vi "Demo.vi"() -> ()   [LabVIEW 2011, in "Mlistbox Tools.lvlib"]
uses:
  Mlistbox Tools.lvlib
  ListBox/Custom Type/Read and Write Mode.ctl
  ListBox/Listbox Tool.lvlib
  Custom Type/Row and Col Option.ctl
panel:
  out "数值显示控件":dbl
  in  "多列列表框":i32(listbox)
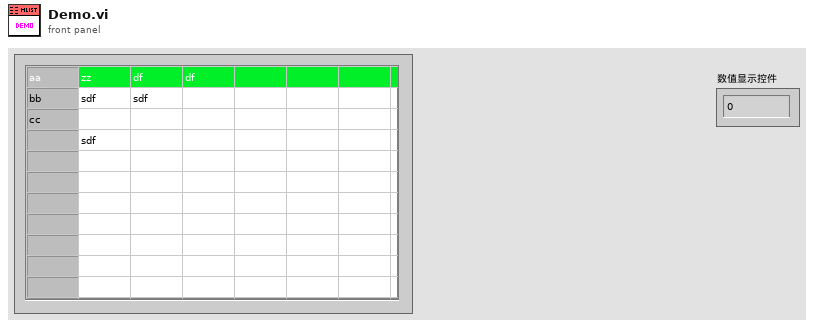
[diagram p1: front panel]
types:
  T1 = typedef "Mlistbox Tools.lvlib/Row and Col Option.ctl" = enum16{"Row", "Col"}
  T2 = typedef "Listbox Tool.lvlib/Read and Write Mode.ctl" = enum16{"Read", "Write"}
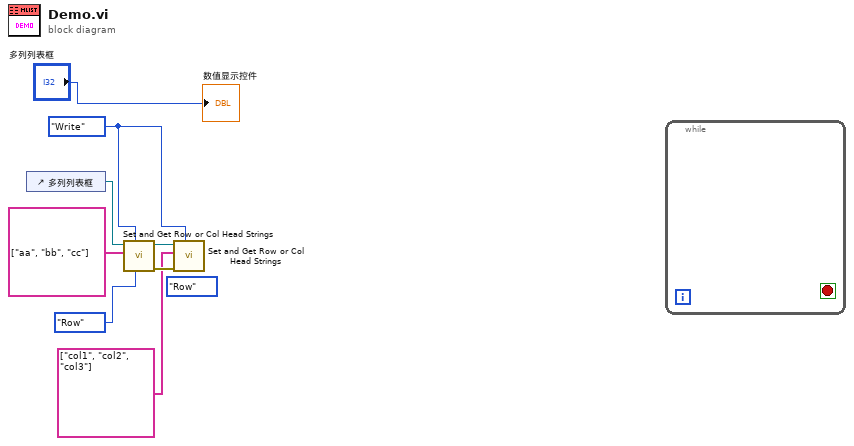
[diagram p0: block diagram]
diagram:
  w2 = Row_and_Col_Option."Row" ("Row Or Col")
  w5 = Read_and_Write_Mode."Write" ("Mode")
  n1 = control-ref of="多列列表框"() -> (w9:refnum<vi>)
  n2 = call "Set and Get Row or Col Head Strings.vi"("Row Or Col"=Row_and_Col_Option."Row", "Mode"=w5, "String[]  In"=string[] ["aa", "bb", "cc"], "Mlistbox Ref"=w9) -> ("错误输出"=w7:errorcluster, "Mlistbox Ref Dup"=w6:refnum<vi>)  [unwired: 5 in, 1 out]
  n3 = call "Set and Get Row or Col Head Strings.vi"("Mode"=w5, "错误输入"=w7, "String[]  In"=string[] ["col1", "col2", "col3"], "Mlistbox Ref"=w6) -> ()  [unwired: 5 in, 3 out]
  n4 = while {
    stop <- _ stop-if-true
  }
  "数值显示控件" <- "多列列表框"
